vi "sealtestwfparams.vi"(0 "command":string="get", 1 "Params in":T1={"AO parameters"=[{"AOtab"=0.0, "Repeats"=1.0, "Cycles"=10.0, "Start amplitude (V)"=0.1, "Baseline (V)"=0.0, "Step size (V)"=0.0, "DC (%)"=50.0, "Sampling frequency (Hz)"=10000.0, "Period (ms)"=10.0, "Offset (V)"=0.0, "Amplitude (V)"=0.0, "Frequency"=0.0, "Tri Repeats"=0.0, "Cycle length (s)"=0.0, "Pulses"=1.0, "Matlab wave file"=path "", "Tri phase"=0.0, "padding value"=0.0}, {"AOtab"=0.0, "Repeats"=1.0, "Cycles"=10.0, "Start amplitude (V)"=0.0, "Baseline (V)"=0.0, "Step size (V)"=0.0, "DC (%)"=0.0, "Sampling frequency (Hz)"=10000.0, "Period (ms)"=10.0, "Offset (V)"=0.0, "Amplitude (V)"=0.0, "Frequency"=0.0, "Tri Repeats"=0.0, "Cycle length (s)"=0.0, "Pulses"=1.0, "Matlab wave file"=path "", "Tri phase"=0.0, "padding value"=0.0}]}) -> (5 "Params out":T1={"AO parameters"=[{"AOtab"=0.0, "Repeats"=1.0, "Cycles"=1.0, "Start amplitude (V)"=0.01, "Baseline (V)"=0.0, "Step size (V)"=0.0, "DC (%)"=50.0, "Sampling frequency (Hz)"=5000.0, "Period (ms)"=10.0, "Offset (V)"=0.0, "Amplitude (V)"=0.0, "Frequency"=0.0, "Tri Repeats"=0.0, "Cycle length (s)"=0.0, "Pulses"=10.0, "Matlab wave file"=path "", "Tri phase"=0.0, "padding value"=0.0}, {"AOtab"=0.0, "Repeats"=1.0, "Cycles"=10.0, "Start amplitude (V)"=0.0, "Baseline (V)"=0.0, "Step size (V)"=0.0, "DC (%)"=0.0, "Sampling frequency (Hz)"=10000.0, "Period (ms)"=10.0, "Offset (V)"=0.0, "Amplitude (V)"=0.0, "Frequency"=0.0, "Tri Repeats"=0.0, "Cycle length (s)"=0.0, "Pulses"=1.0, "Matlab wave file"=path "", "Tri phase"=0.0, "padding value"=0.0}]})   [LabVIEW 2015]
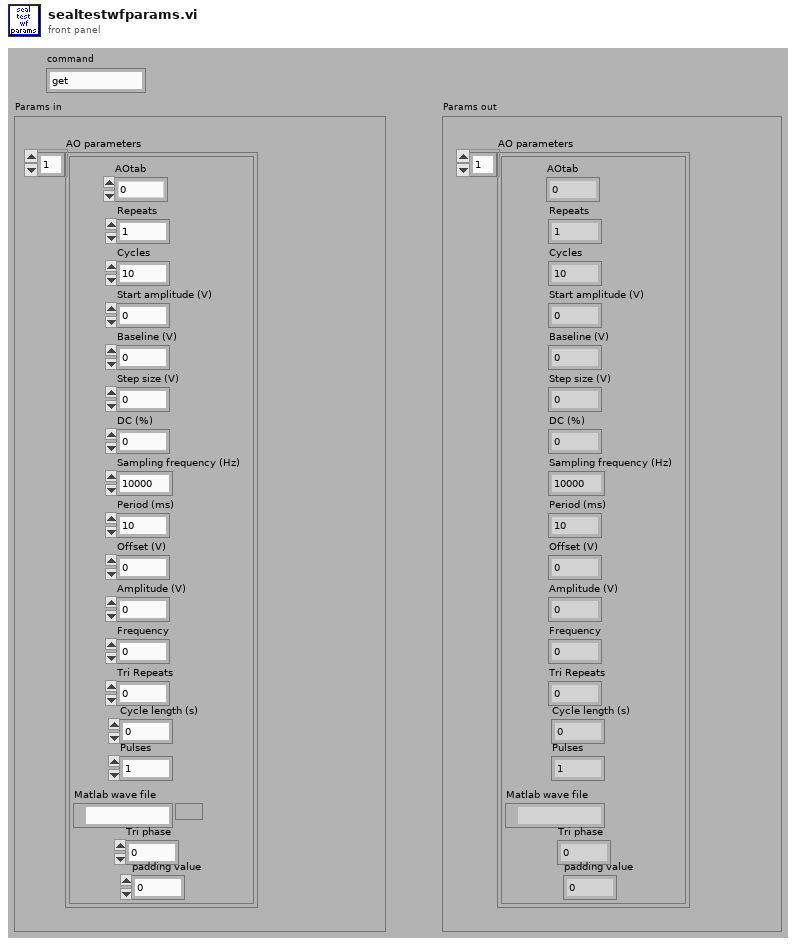
[diagram p1: front panel]
types:
  T1 = cluster{"AO parameters":cluster{"AOtab":dbl, "Repeats":dbl, "Cycles":dbl, "Start amplitude (V)":dbl, "Baseline (V)":dbl, "Step size (V)":dbl, "DC (%)":dbl, "Sampling frequency (Hz)":dbl, "Period (ms)":dbl, "Offset (V)":dbl, "Amplitude (V)":dbl, "Frequency":dbl, "Tri Repeats":dbl, "Cycle length (s)":dbl, "Pulses":dbl, "Matlab wave file":path, "Tri phase":dbl, "padding value":dbl}[]}
  T2 = cluster{"AOtab":dbl, "Repeats":dbl, "Cycles":dbl, "Start amplitude (V)":dbl, "Baseline (V)":dbl, "Step size (V)":dbl, "DC (%)":dbl, "Sampling frequency (Hz)":dbl, "Period (ms)":dbl, "Offset (V)":dbl, "Amplitude (V)":dbl, "Frequency":dbl, "Tri Repeats":dbl, "Cycle length (s)":dbl, "Pulses":dbl, "Matlab wave file":path, "Tri phase":dbl, "padding value":dbl}[]
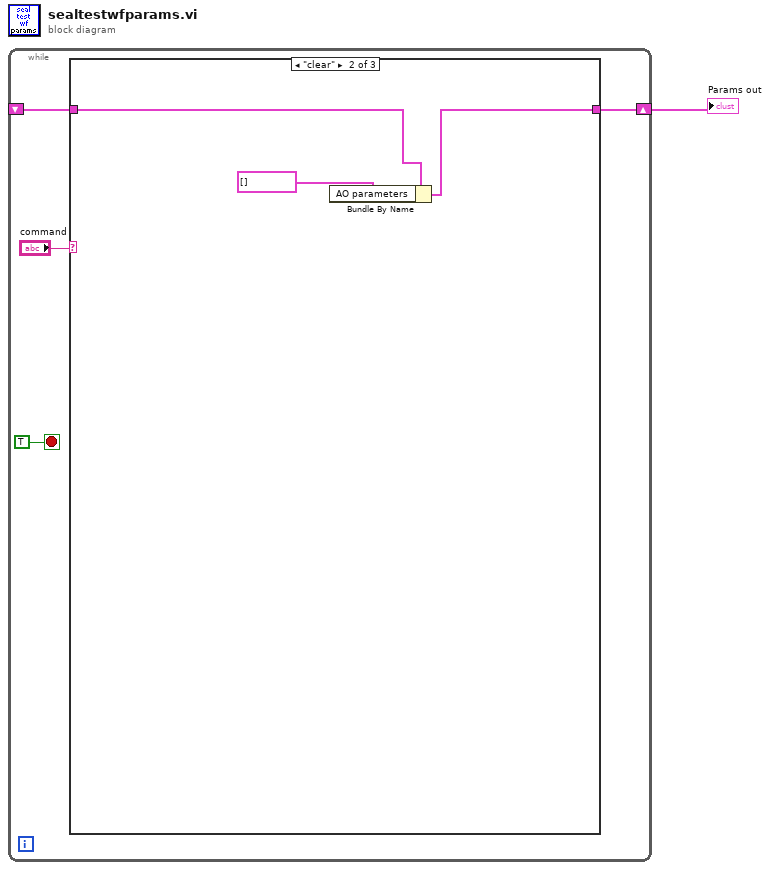
[diagram p0: block diagram]
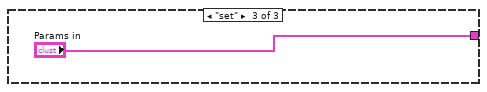
[diagram p3: hidden frame]
diagram:
  n1 = while {
    shift-right: [w3] -> w1
    shift-left: _ -> [w2]
    stop <- TRUE stop-if-true
    n2 = case shown="\"clear\"" "command" {
      tunnel: [w6 w8 "Params in"] -> w3
      tunnel: w2 -> [w6 w9 _]
      frame "get", Default {
      }
      frame "clear" {
        n3 = Bundle By Name(cluster=w9, "AO parameters"=T2 []) -> (w8:T1)
      }
      frame "set" {
      }
    }
  }
  "Params out" <- w1
